vi "TR_UNIT_ARR_2_STR_ARR.vi"(1 "offset":i32, 7 "TR_Unit_Arr":T1[](array[typedef]), 12 "format":enum16{"hex", "dec", "oct", "bin"}(ring), 14 "TSFormat":enum16{"原始值", "实际值"}(ring)) -> (3 "smb":i32[](array[numeric]), 8 "strTable":string[][](array[string]))   [LabVIEW 2011]
uses:
  _USB_CAN_T_R_Unit_.ctl
  _USB_CAN_GLOBAL_.vi
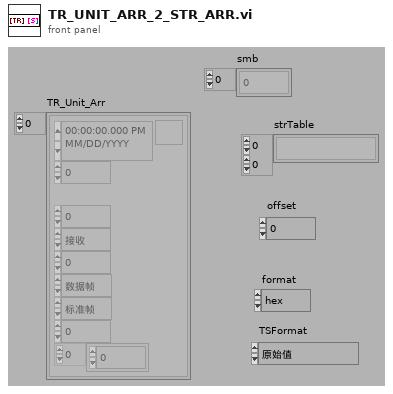
[diagram p1: front panel]
types:
  T1 = typedef "_USB_CAN_T_R_Unit_.ctl" = cluster{"time":timestamp, "channel":u16, "TimeStamp":u32, "tr":enum16{"接收", "发送"}, "id":u32, "Type":enum16{"数据帧", "远程帧"}, "Format":enum16{"标准帧", "扩展帧"}, "len":u8, "data":u8[]}
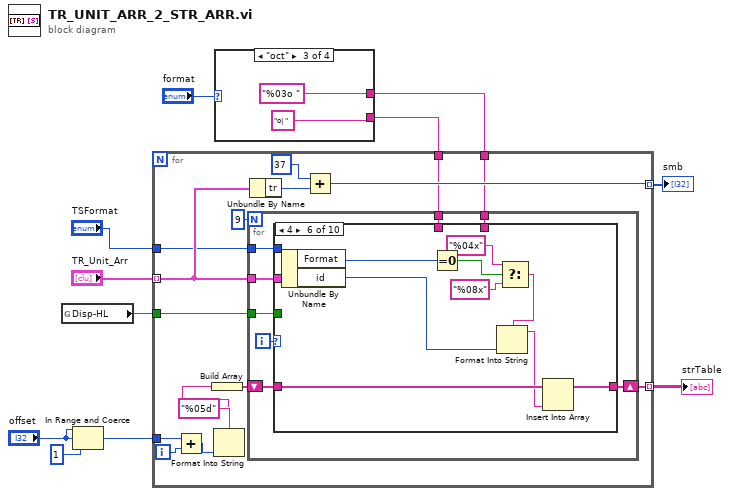
[diagram p0: block diagram]
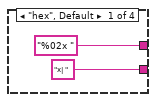
[diagram p2: hidden frame]
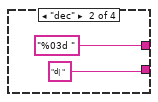
[diagram p3: hidden frame]
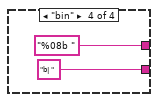
[diagram p4: hidden frame]
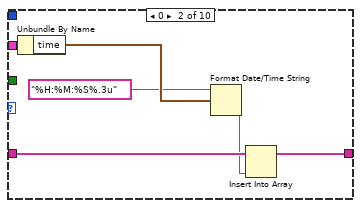
[diagram p6: hidden frame]
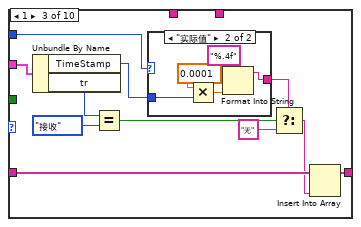
[diagram p7: hidden frame]
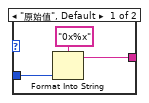
[diagram p8: hidden frame]
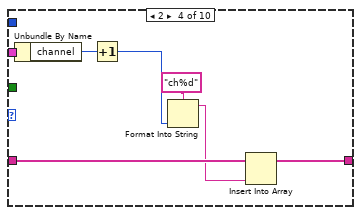
[diagram p9: hidden frame]
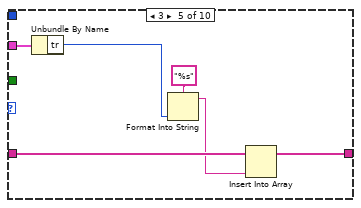
[diagram p10: hidden frame]
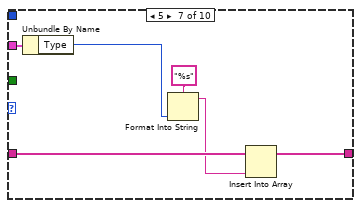
[diagram p11: hidden frame]
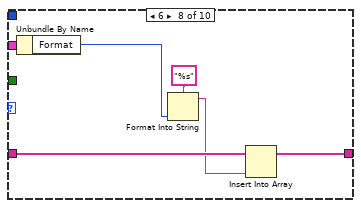
[diagram p12: hidden frame]
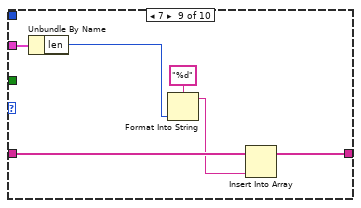
[diagram p13: hidden frame]
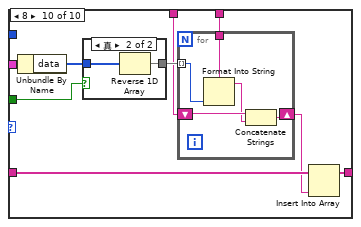
[diagram p14: hidden frame]
diagram:
  n1 = global read "_USB_CAN_GLOBAL_.vi" "Disp-HL"() -> (w8:bool)
  n2 = In Range and Coerce(upper limit="offset", x="offset", lower limit=1 ("下限")) -> (coerced(x)=w4:i32)  [unwired: 1 out]
  n3 = case shown="\"oct\"" "format" {
    tunnel: ["%02x " ("格式字符串") "%03d " ("格式字符串") "%03o " ("格式字符串") "%08b " ("格式字符串")] -> w6
    tunnel: ["x| " ("格式字符串") "d| " ("格式字符串") "o| " ("格式字符串") "b| " ("格式字符串")] -> w5
    frame "hex", Default {
    }
    frame "dec" {
    }
    frame "oct" {
    }
    frame "bin" {
    }
  }
  n4 = for {
    tunnel: "TR_Unit_Arr" -> [w27] mode=indexing
    tunnel: [w31] -> w11 mode=indexing
    tunnel: w4 -> [w29]
    tunnel: [w24] -> w9 mode=indexing
    tunnel: w8 -> [w23]
    tunnel: w6 -> [w22]
    tunnel: w5 -> [w21]
    tunnel: "TSFormat" -> [w20]
    i -> [w30]
    n5 = Add(x=w29, y=w30) -> (x+y=w28:i32)
    n6 = Format Into String(format string="%05d" ("格式字符串"), w28) -> (resulting string=w34:string)  [unwired: 2 in, 1 out]
    n7 = Build Array(w34) -> (w33:string[])
    n8 = for {
      N: 9 -> [_]
      shift-right: [w40] -> w31
      shift-left: w33 -> [w42]
      tunnel: w27 -> [w41]
      tunnel: w23 -> [w39]
      tunnel: w22 -> [w38]
      tunnel: w21 -> [w37]
      tunnel: w20 -> [w36]
      i -> [w43]
      n9 = case shown="4" w43 {
        tunnel: w42 -> [w44 w47 w60 w75 w81 w91 w97 w103 w109 w118]
        tunnel: w41 -> [_ w50 w61 w76 w82 w92 w98 w104 w110 w119]
        tunnel: [w44 w45 w59 w74 w80 w90 w96 w102 w108 w117] -> w40
        tunnel: w39 -> [_ _ _ _ _ _ _ _ _ w113]
        tunnel: w38 -> [_ _ _ _ _ _ _ _ _ w112]
        tunnel: w37 -> [_ _ _ _ _ _ _ _ _ w111]
        tunnel: w36 -> [_ _ w51 _ _ _ _ _ _ _]
        frame -1, Default {
        }
        frame 0 {
          n10 = Unbundle By Name(w50) -> ("time"=w49:timestamp)
          n11 = Format Date/Time String(time format string (%c)="%H:%M:%S%.3u" ("时间格式字符串(%c)"), seconds (now)=w49) -> (date/time string=w46:string)  [unwired: 1 in]
          n12 = Insert Into Array(array=w47, new element=w46) -> (w45:string[])  [unwired: 1 in]
        }
        frame 1 {
          n13 = Unbundle By Name(w61) -> ("TimeStamp"=w55:u32, "tr"=w58:enum16{"接收", "发送"})
          n14 = Equal?(x=w58, y=enum16{"接收", "发送"}."接收") -> (x = y?=w56:bool)
          n15 = case shown="\"实际值\"" w51 {
            tunnel: w55 -> [w64 w69]
            tunnel: [w62 w65] -> w54
            frame "原始值", Default {
              n16 = Format Into String(format string="0x%x" ("格式字符串"), w64) -> (resulting string=w62:string)  [unwired: 2 in, 1 out]
            }
            frame "实际值" {
              n17 = Multiply(x=0.0001, y=w69) -> (x*y=w67:dbl)
              n18 = Format Into String(format string="%.4f" ("格式字符串"), w67) -> (resulting string=w65:string)  [unwired: 2 in, 1 out]
            }
          }
          n19 = Select(t=w54, s=w56, f="无") -> (s? t:f=w52:string)
          n20 = Insert Into Array(array=w60, new element=w52) -> (w59:string[])  [unwired: 1 in]
        }
        frame 2 {
          n21 = Unbundle By Name(w76) -> ("channel"=w73:u16)
          n22 = Increment(x=w73) -> (x+1=w70:u16)
          n23 = Format Into String(format string="ch%d" ("格式字符串"), w70) -> (resulting string=w72:string)  [unwired: 2 in, 1 out]
          n24 = Insert Into Array(array=w75, new element=w72) -> (w74:string[])  [unwired: 1 in]
        }
        frame 3 {
          n25 = Unbundle By Name(w82) -> ("tr"=w79:enum16{"接收", "发送"})
          n26 = Format Into String(format string="%s" ("格式字符串"), w79) -> (resulting string=w78:string)  [unwired: 2 in, 1 out]
          n27 = Insert Into Array(array=w81, new element=w78) -> (w80:string[])  [unwired: 1 in]
        }
        frame 4 {
          n28 = Unbundle By Name(w92) -> ("Format"=w87:enum16{"标准帧", "扩展帧"}, "id"=w89:u32)
          n29 = Equal To 0?(x=w87) -> (x = 0?=w86:bool)
          n30 = Select(t="%04x" ("格式字符串"), s=w86, f="%08x" ("格式字符串")) -> (s? t:f=w83:string)
          n31 = Format Into String(format string=w83, w89) -> (resulting string=w88:string)  [unwired: 2 in, 1 out]
          n32 = Insert Into Array(array=w91, new element=w88) -> (w90:string[])  [unwired: 1 in]
        }
        frame 5 {
          n33 = Unbundle By Name(w98) -> ("Type"=w95:enum16{"数据帧", "远程帧"})
          n34 = Format Into String(format string="%s" ("格式字符串"), w95) -> (resulting string=w94:string)  [unwired: 2 in, 1 out]
          n35 = Insert Into Array(array=w97, new element=w94) -> (w96:string[])  [unwired: 1 in]
        }
        frame 6 {
          n36 = Unbundle By Name(w104) -> ("Format"=w101:enum16{"标准帧", "扩展帧"})
          n37 = Format Into String(format string="%s" ("格式字符串"), w101) -> (resulting string=w100:string)  [unwired: 2 in, 1 out]
          n38 = Insert Into Array(array=w103, new element=w100) -> (w102:string[])  [unwired: 1 in]
        }
        frame 7 {
          n39 = Unbundle By Name(w110) -> ("len"=w107:u8)
          n40 = Format Into String(format string="%d" ("格式字符串"), w107) -> (resulting string=w106:string)  [unwired: 2 in, 1 out]
          n41 = Insert Into Array(array=w109, new element=w106) -> (w108:string[])  [unwired: 1 in]
        }
        frame 8 {
          n42 = Unbundle By Name(w119) -> ("data"=w116:u8[])
          n43 = case shown="真" w113 {
            tunnel: w116 -> [w120 w122]
            tunnel: [w120 w121] -> w114
            frame False {
            }
            frame True {
              n44 = Reverse 1D Array(array=w122) -> (reversed array=w121:u8[])
            }
          }
          n45 = for {
            tunnel: w114 -> [w127] mode=indexing
            shift-right: [w126] -> w115
            shift-left: w111 -> [w125]
            tunnel: w112 -> [w123]
            n46 = Format Into String(format string=w123, w127) -> (resulting string=w124:string)  [unwired: 2 in, 1 out]
            n47 = Concatenate Strings(w125, w124) -> (w126:string)
          }
          n48 = Insert Into Array(array=w118, new element=w115) -> (w117:string[])  [unwired: 1 in]
        }
      }
    }
    n49 = Unbundle By Name(w27) -> ("tr"=w26:enum16{"接收", "发送"})
    n50 = Add(x=37, y=w26) -> (x+y=w24:i32)
  }
  "strTable" <- w11
  "smb" <- w9
